vi "실습 7-1.vi"() -> ()   [LabVIEW 2014]
uses:
  kernel32.dll
panel:
  out "Current Process ID":i32
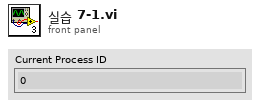
[diagram p1: front panel]
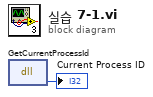
[diagram p0: block diagram]
diagram:
  n1 = dll-call lib="kernel32.dll" fn="GetCurrentProcessId"() -> ("반환 타입"=→"Current Process ID":i32)  [unwired: 3 in, 2 out]
